vi "OCR_Seperate rectangle into bit array.vi"(8 "Error":errorcluster, 9 "Text Rect.":T2={"window"={"Left"=0, "Top"=0, "Right"=0, "Bottom"=0, "Width"=0, "Height"=0, "Start"={"Left"=0, "Top"=0}}, "Color"={"BG"=16776960, "FG"=255}, "Status"=FALSE}, 11 "2D Image":T1) -> (0 "Error Out":errorcluster, 3 "Bit Array Out":T6)   [LabVIEW 2009]
doc: "Seperates out a Line of text into an array of bit arrays"
uses:
  Controls/Cluster/Cluster_Bit array and line status.ctl
  Controls/String_Picture/String Char Normal.ctl
  Controls/Cluster/Cluster_Text Rect.ctl
  Controls/Cluster/Cluster_Region info.ctl
  Controls/Cluster/Cluster_Top Left position.ctl
  Controls/Cluster/Cluster_Text Color Set.ctl
  Controls/Array/Color Box Array_2D Icon Viewer.ctl
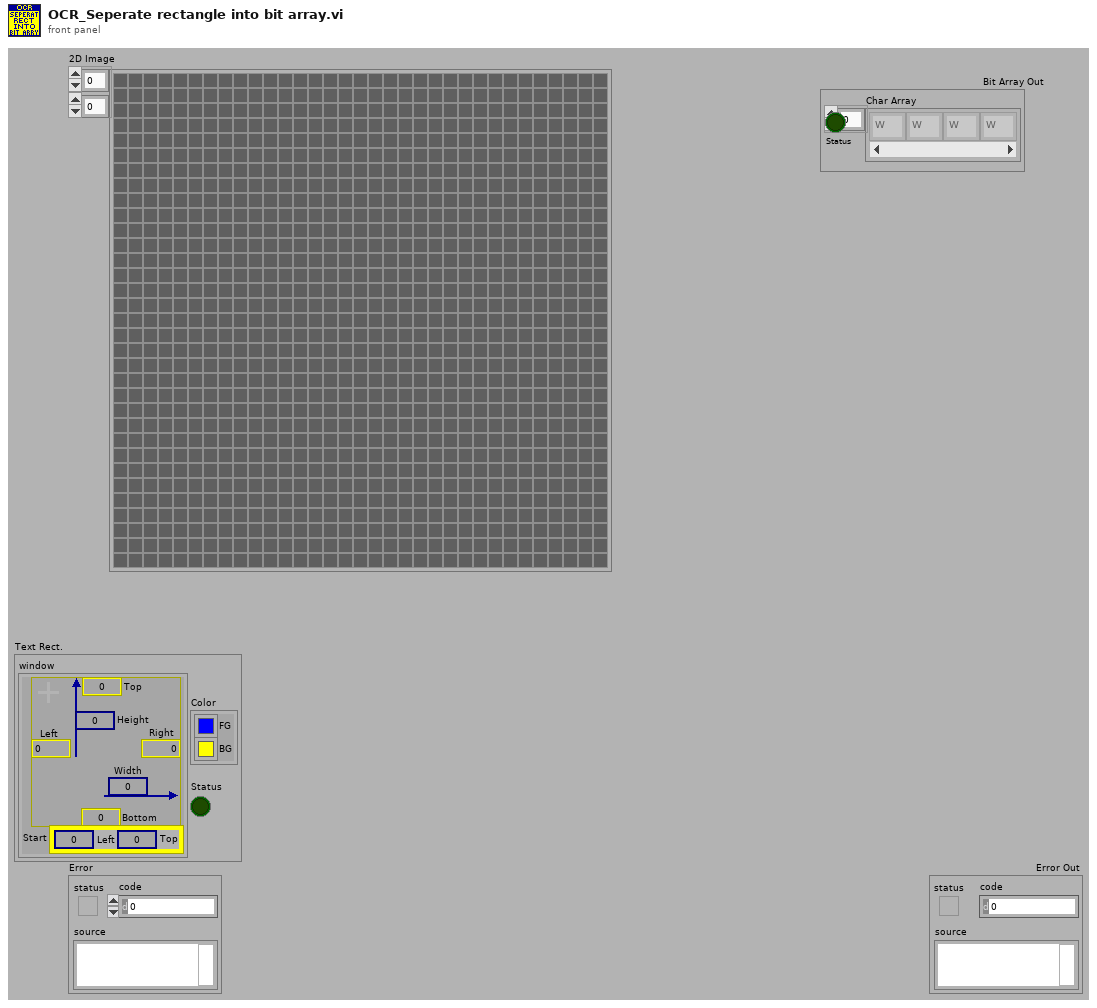
[diagram p1: front panel]
types:
  T1 = typedef "Color Box Array_2D Icon Viewer.ctl" = u32[][]
  T2 = typedef "Cluster_Text Rect.ctl" = cluster{"window":T3, "Color":T5, "Status":bool}
  T3 = typedef "Cluster_Region info.ctl" = cluster{"Left":i32, "Top":i32, "Right":i32, "Bottom":i32, "Width":u32, "Height":u32, "Start":T4}
  T4 = typedef "Cluster_Top Left position.ctl" = cluster{"Left":i32, "Top":i32}
  T5 = typedef "Cluster_Text Color Set.ctl" = cluster{"BG":u32, "FG":u32}
  T6 = typedef "Cluster_Bit array and line status.ctl" = cluster{"Char Array":T7[], "Status":bool}
  T7 = typedef "String Char Normal.ctl" = string
  T8 = typedef "ENUM_Line Letter Type.ctl" = enum16{"Unknown", "Letter", "Seperator", "Seperator or Letter"}
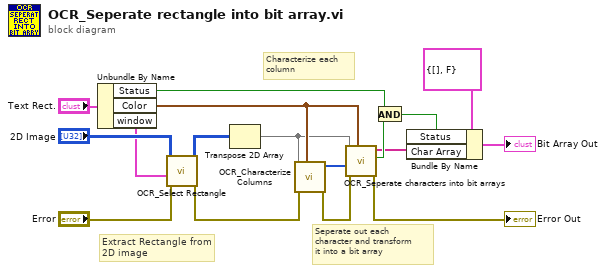
[diagram p0: block diagram]
diagram:
  # "Seperate out each\ncharacter and transform\nit into a bit array"
  # "Characterize each\ncolumn"
  # "Extract Rectangle from\n2D image"
  n1 = Unbundle By Name("Text Rect.") -> ("Status"=w8:bool, "Color"=w10:T5, "window"=w2:T3)
  n2 = call "OCR_Select Rectangle.vi"("Error"="Error", "Region"=w2, "2D Image"="2D Image") -> ("Error Out"=w14:errorcluster, "2D Image Out"=w4:T1)  [unwired: 7 in]
  n3 = Transpose 2D Array(2D array=w4) -> (transposed array=w3:T1)
  n4 = call "OCR_Characterize Columns.vi"("Color Set"=w10, "Error"=w14, "2D Image"=w3) -> ("Error Out"=w15:errorcluster, "Column Type Aray Out"=w17:T8[])  [unwired: 7 in]
  n5 = call "OCR_Seperate characters into bit arrays.vi"("Color Set"=w10, "Error"=w15, "Column Type Array"=w17, "2D Image"=w3) -> ("Error Out"=→"Error Out":errorcluster, "All Good Out"=w9:bool, "Char Array Out"=w1:T7[])  [unwired: 5 in]
  n6 = And(x=w8, y=w9) -> (x .and. y?=w5:bool)
  n7 = Bundle By Name(cluster=T6 {"Char Array"=[], "Status"=FALSE} ("Bit Array Out"), "Status"=w5, "Char Array"=w1) -> (→"Bit Array Out":T6)
